vi "Set Magnet Field.vi"(4 "Mode":T2, 6 "Axis":T1, 8 "error in (no error)":errorcluster, 9 "Target Rate (T/min)":dbl, 10 "Target Field (T)":dbl, 11 "Instrument.Oxford1820 in":refnum<class "Instrument.Oxford1820.lvclass">) -> (0 "error out":errorcluster, 3 "Instrument.Oxford1820 out":refnum<class "Instrument.Oxford1820.lvclass">)   [LabVIEW 2016, in "Instrument.Oxford1820.lvclass"]
uses:
  Instrument.Oxford1820.lvclass
  <userlib>/LevyLab/Levylab Instruments/Instrument Types/Cryostat/Typedefs/Magnet Mode--Enum.ctl
  <userlib>/LevyLab/Levylab Instruments/Instrument Types/Cryostat/Typedefs/Magnet Axis--Enum.ctl
  Typedefs/Targets.ctl
  <userlib>/LevyLab/Levylab Instruments/Instrument Types/Cryostat/Instrument.Cryostat.lvclass
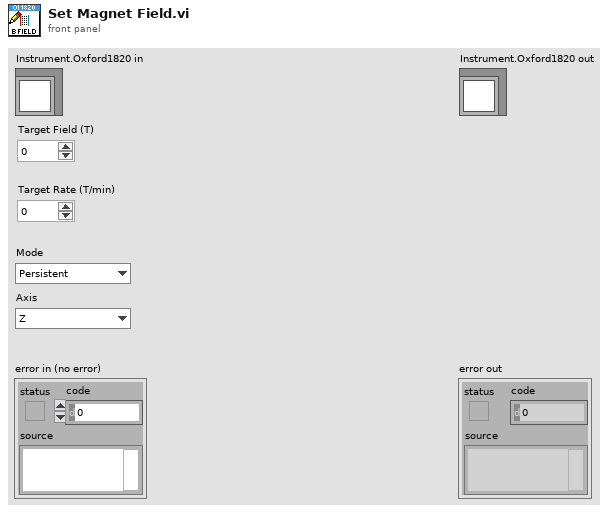
[diagram p1: front panel]
types:
  T1 = typedef "Instrument.Cryostat.lvclass/Magnet Axis--Enum.ctl" = enum16{"Z", "X", "Y"}
  T2 = typedef "Instrument.Cryostat.lvclass/Magnet Mode--Enum.ctl" = enum16{"Persistent", "Driven"}
  T3 = typedef "Instrument.Oxford1820.lvclass/Targets.ctl" = cluster{"Target Field (T)":dbl, "Target Field Rate (T/min)":dbl}
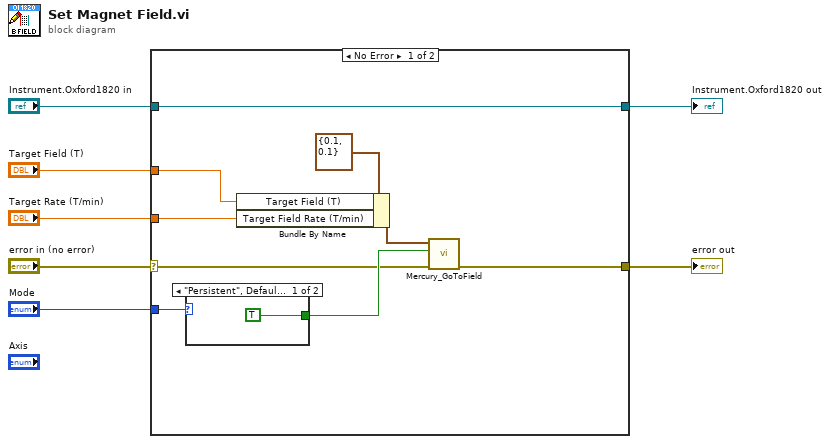
[diagram p0: block diagram]
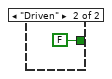
[diagram p2: hidden frame]
diagram:
  n1 = case shown="No Error" "error in (no error)" {
    selector: "error in (no error)" -> [w9 w20]
    tunnel: "Mode" -> [w16 _]
    tunnel: "Target Rate (T/min)" -> [w15 _]
    tunnel: [w8 w20] -> w5
    tunnel: "Target Field (T)" -> [w13 _]
    tunnel: "Instrument.Oxford1820 in" -> [w12 w19]
    tunnel: [w12 w19] -> w1
    frame No Error {
      n2 = case shown="\"Persistent\", Default" w16 {
        tunnel: [TRUE ("persistent mode") FALSE ("persistent mode")] -> w10
        frame "Persistent", Default {
        }
        frame "Driven" {
        }
      }
      n3 = Bundle By Name(cluster=T3 {"Target Field (T)"=0.1, "Target Field Rate (T/min)"=0.1} ("Mercury Targets"), "Target Field (T)"=w13, "Target Field Rate (T/min)"=w15) -> (w11:T3)
      n4 = call "Mercury_GoToField.vi"("error in"=w9, "persistent mode"=w10, "Mercury Targets"=w11) -> ("error out"=w8:errorcluster)  [unwired: 8 in]
    }
    frame Error {
    }
  }
  "Instrument.Oxford1820 out" <- w1
  "error out" <- w5
